vi "RunTestsCore.vi"(8 "error in (no error)":errorcluster) -> (0 "error out":errorcluster)   [LabVIEW 2016, in "Drona.lvlib"]
uses:
  Drona.lvlib
  Stimulus/VI/RunVI.vi
  <vilib>/Utility/LVLibp/NI_PackedLibraryUtility.lvlib
  <vilib>/addons/_JKI Toolkits/Caraya/classes/Test/Test.lvclass
  Stimulus/VI/VI.lvlib
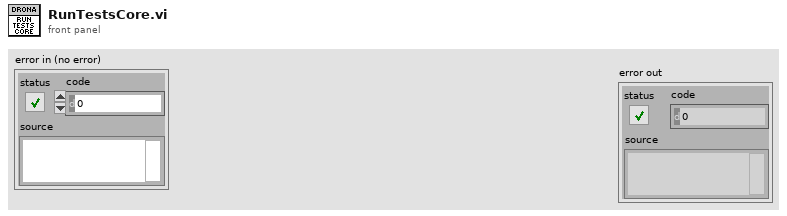
[diagram p1: front panel]
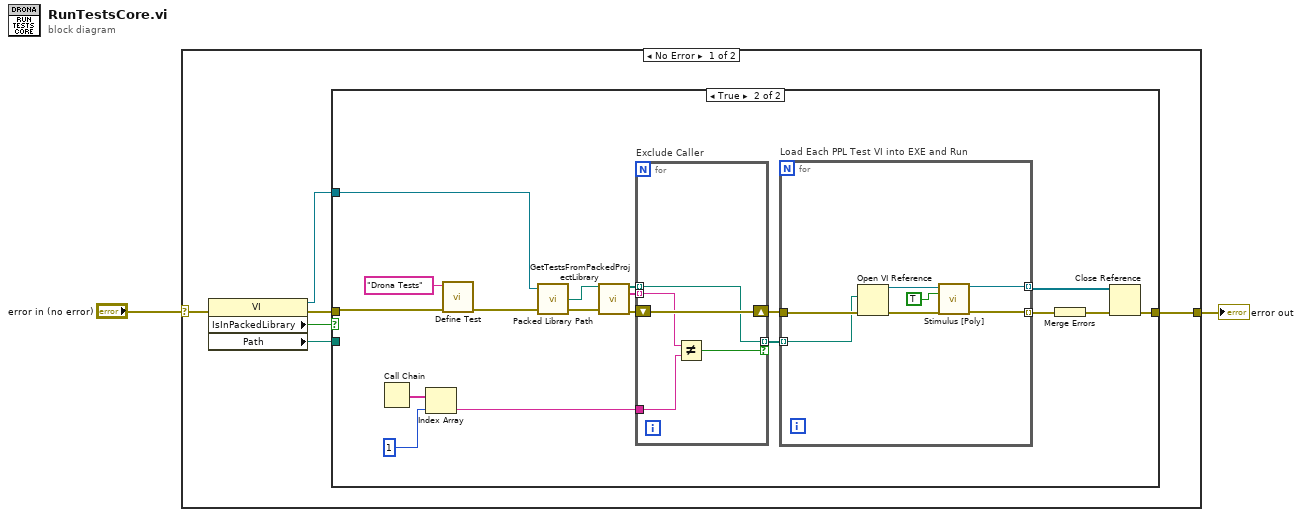
[diagram p0: block diagram]
diagram:
  n1 = case shown="No Error" "error in (no error)" {
    selector: "error in (no error)" -> [w8 w40]
    tunnel: [w4 w40] -> w2
    frame No Error {
      n2 = property class="VI"(error in=w8) -> (reference out=w5:refnum<vi>, error out=w7:errorcluster, "IsInPackedLibrary"=w6:bool, "Path"=w3:path)  [unwired: 1 in]
      n3 = case shown="True" w6 {
        tunnel: w7 -> [w9 w25]
        tunnel: w5 -> [_ w24]
        tunnel: [w9 w21] -> w4
        tunnel: w3 -> [_ _]
        frame False {
        }
        frame True {
          n4 = Call Chain() -> (call chain=w10:string[])
          n5 = Index Array(array=w10, index=1) -> (element=w11:string)
          n6 = call <vilib>:"Define Test.vi"("error in (no error)"=w25, "Label (VI Title)"="Drona Tests") -> ("error out"=w20:errorcluster)  [unwired: 9 in]
          n7 = call <vilib>:"Packed Library Path.vi"("error in (no error)"=w20, "vi reference"=w24) -> ("error out"=w22:errorcluster, "packed library path"=w23:path)  [unwired: 1 in, 1 out]
          n8 = call "GetTestsFromPackedProjectLibrary.vi"("Packed Project Library Path"=w23, "error in (no error)"=w22) -> ("Tests"=w17:path[], "Qualified Names"=w12:string[], "error out"=w16:errorcluster)  [unwired: 11 in]
          n9 = for "Exclude Caller" {
            tunnel: w17 -> [w28] mode=indexing
            tunnel: [w28] -> w15 mode=indexing if=w32
            shift-right: [w31] -> w14
            shift-left: w16 -> [w31]
            tunnel: w12 -> [w30] mode=indexing
            tunnel: w11 -> [w29]
            n10 = Not Equal?(x=w30, y=w29) -> (x != y?=w32:bool)
          }
          n11 = for "Load Each PPL Test VI into EXE and Run" {
            tunnel: w15 -> [w34] mode=indexing
            tunnel: [w37] -> w26 mode=indexing
            tunnel: w14 -> [w36]
            tunnel: [w39] -> w27 mode=indexing
            n12 = Open VI Reference(vi path=w34, error in (no error)=w36) -> (vi reference=w33:refnum<vi>, error out=w35:errorcluster)  [unwired: 4 in]
            n13 = call-poly "Stimulus [Poly].vi"("VI Reference In"=w33, "Wait Until Done (F)"=TRUE, "error in"=w35) -> ("VI Reference Out"=w37:refnum<vi>, "error out"=w39:errorcluster)  [unwired: 11 in]
          }
          n14 = Merge Errors(w27) -> (w18:errorcluster)
          n15 = Close Reference(reference=w26, error in (no error)=w18) -> (error out=w21:errorcluster)
        }
      }
    }
    frame Error {
    }
  }
  "error out" <- w2
